vi "Power_Tunings_Tester_Parameter.vi"() -> (3 "Power_Tuning_Tester_Parameter":dbl[](array[numeric]))   [LabVIEW 2017]
panel:
  out "all":string
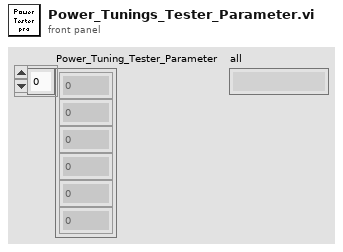
[diagram p1: front panel]
types:
  T1 = typedef "HD Config.ctl" = cluster{" PC":cluster{"PC Address":u8[], "PC Port":i32}, "FCO":cluster{"COM":refnum<visa-resource-name>, "Baudrate":u32}, "DC Power ":cluster{"COM":refnum<visa-resource-name>, "Baudrate":u32}, "PW3336":cluster{"COM":refnum<visa-resource-name>, "Baudrate":u32}, "Lefoo":cluster{"COM":refnum<visa-resource-name>, "Baudrate":u32}, "Tempt&Hum":cluster{"COM":refnum<visa-resource-name>, "Baudrate":u32}, "DIPC":cluster{"COM":refnum<visa-resource-name>}, "Daemon":cluster{"IP Address":string, "Port":u16, "Retry":u16}, "Motor":cluster{"COM":refnum<visa-resource-name>, "Baudrate":u32}, "Fail_resume_mode":bool, "GRR":bool}
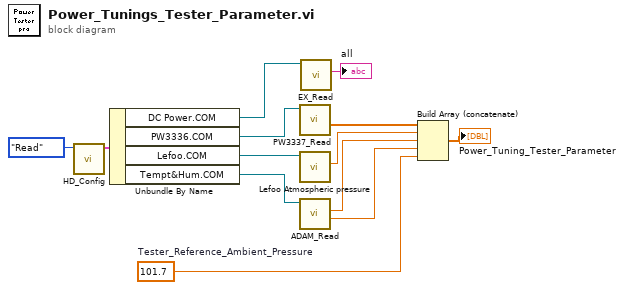
[diagram p0: block diagram]
diagram:
  w6 = 101.7  # Tester_Reference_Ambient_Pressure
  n1 = call "HD_Config.vi"("Step"=enum16{"Initial", "Write", "Read"}."Read") -> ("HD Config out"=w12:T1)  [unwired: 9 in, 1 out]
  n2 = Unbundle By Name(w12) -> ("DC Power.COM"=w2:refnum<visa-resource-name>, "PW3336.COM"=w11:refnum<visa-resource-name>, "Lefoo.COM"=w10:refnum<visa-resource-name>, "Tempt&Hum.COM"=w9:refnum<visa-resource-name>)
  n3 = call "PW3337_Read.vi"("VISA resource name"=w11) -> ("Measurement out"=w8:dbl[])  [unwired: 7 in, 3 out]
  n4 = call "Lefoo Atmospheric pressure.vi"("VISA resource name"=w10) -> ("Atmospheric pressure"=w7:dbl)  [unwired: 8 in, 2 out]
  n5 = call "ADAM_Read.vi"("VISA resource name"=w9) -> ("humidity"=w3:dbl, "temperature"=w4:dbl)  [unwired: 7 in, 2 out]
  n6 = call "EX_Read.vi"("VISA resource name"=w2) -> ("读取缓冲区"=→"all":string)  [unwired: 8 in, 2 out]
  n7 = Build Array (concatenate)(w8, w7, w4, w3, w6) -> (→"Power_Tuning_Tester_Parameter":dbl[])
